vi "Get Image Strip subset.vi"(6 "Horizontal?":bool, 7 "Subset Width (100 pixels)":i32=100, 8 "error in":errorcluster, 9 "Dest Image":T1, 10 "Center Pixel (-1)":i32=-1, 11 "Source Image":T1) -> (0 "error out":errorcluster, 3 "Subset out":T1)   [LabVIEW 2009]
doc: "Reentrant\nGet image subset from middle (Width input )pixels and copy into the destination buffer"
uses:
  <vilib>/vision/Image Controls.llb/IMAQ Image.ctl
  <vilib>/vision/NI_Vision_Development_Module.lvlib
panel:
  # "-1 == Use center of image"
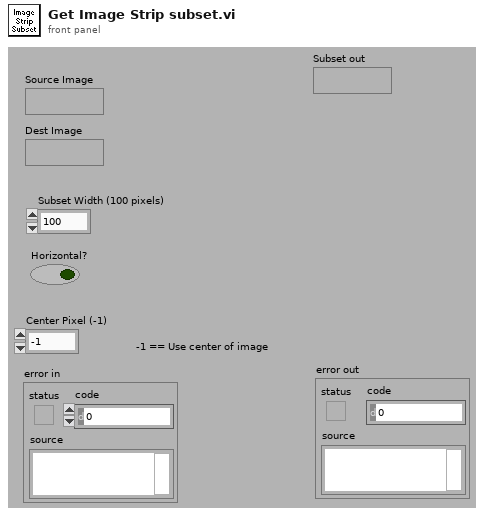
[diagram p1: front panel]
types:
  T1 = typedef "IMAQ Image.ctl" = refnum<image>
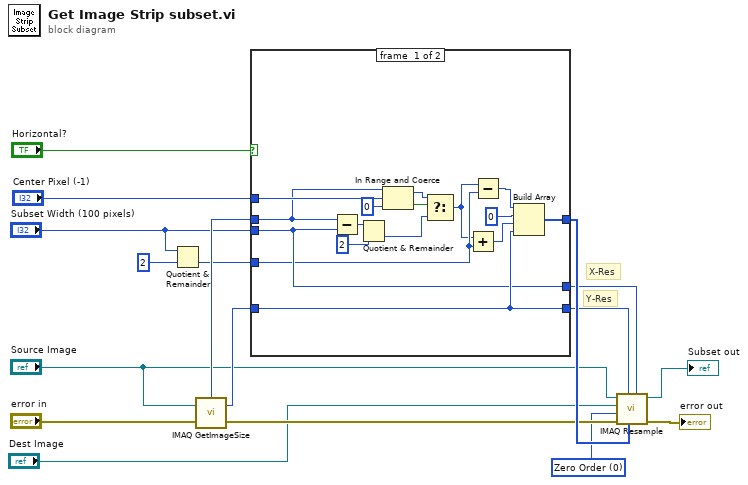
[diagram p0: block diagram]
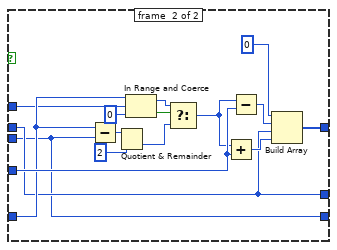
[diagram p2: hidden frame]
diagram:
  w5 = u32 0 items=["Zero Order", "Bi-Linear", "Quadratic", "Cubic Spline"] ("Interpolation Type")
  # "Y-Res"
  # "X-Res"
  n1 = Quotient & Remainder(x="Subset Width (100 pixels)", y=2) -> (floor(x/y)=w2:i32)  [unwired: 1 out]
  n2 = call "IMAQ GetImageSize"("Image"="Source Image", "error in (no error)"="error in") -> ("Y Resolution"=w17:i32, "X Resolution"=w15:i32, "error out"=w14:errorcluster)  [unwired: 2 out]
  n3 = case shown="False" "Horizontal?" {
    tunnel: "Subset Width (100 pixels)" -> [w28 w34]
    tunnel: w17 -> [w29 w39]
    tunnel: [w33 w49] -> w16
    tunnel: w15 -> [w23 w35]
    tunnel: [w29 w34] -> w7
    tunnel: [w28 w35] -> w6
    tunnel: w2 -> [w26 w45]
    tunnel: "Center Pixel (-1)" -> [w24 w38]
    frame #0 {
      n4 = Subtract(x=w23, y=w28) -> (x-y=w30:i32)
      n5 = Quotient & Remainder(x=w30, y=2) -> (floor(x/y)=w18:i32)  [unwired: 1 out]
      n6 = In Range and Coerce(upper limit=w23, x=w24, lower limit=0) -> (coerced(x)=w20:i32, In Range?=w21:bool)
      n7 = Select(t=w20, s=w21, f=w18) -> (s? t:f=w19:i32)
      n8 = Add(x=w19, y=w26) -> (x+y=w27:i32)
      n9 = Subtract(x=w19, y=w26) -> (x-y=w25:i32)
      n10 = Build Array(w25, 0 ("element"), w27, w29) -> (w33:i32[])
    }
    frame #1 {
      n11 = Subtract(x=w39, y=w34) -> (x-y=w47:i32)
      n12 = Quotient & Remainder(x=w47, y=2) -> (floor(x/y)=w37:i32)  [unwired: 1 out]
      n13 = In Range and Coerce(upper limit=w39, x=w38, lower limit=0) -> (coerced(x)=w42:i32, In Range?=w41:bool)
      n14 = Select(t=w42, s=w41, f=w37) -> (s? t:f=w36:i32)
      n15 = Add(x=w36, y=w45) -> (x+y=w46:i32)
      n16 = Subtract(x=w36, y=w45) -> (x-y=w44:i32)
      n17 = Build Array(0 ("element"), w44, w35, w46) -> (w49:i32[])
    }
  }
  n18 = call "IMAQ Resample"("X Resolution"=w6, "Optional Rectangle"=w16, "Y Resolution"=w7, "error in (no error)"=w14, "Interpolation Type"=w5, "Image Dst"="Dest Image", "Image Src"="Source Image") -> ("error out"=→"error out":errorcluster, "Image Dst Out"=→"Subset out":T1)  [unwired: 3 out]
